vi "Get_Target_Type.vi"(8 "error in (no error)":errorcluster, 9 "install path":string, 10 "default install path":string, 11 "IB_Destination in":refnum<class "IB_Destination.lvclass">) -> (0 "error out":errorcluster, 1 "path for target type":T1=68 items=["Relative to default installation directory"=68, "Root directory on first partition"=70, "Relative to directory table key"=82, "Absolute path to file"=65], 2 "path for target":string, 3 "IB_Destination out":refnum<class "IB_Destination.lvclass">)   [LabVIEW 2020, in "IB_Destination.lvclass"]
uses:
  <vilib>/AppBuilder/IB_Classes/Destination/IB_Destination.lvclass
  <vilib>/AppBuilder/IB_Classes/Destination/IB_Destination.lvclass/IB_Destination.ctl
  AppLibs/distkit/MDF/NIMdf.llb/MDFBDPAddFilePathType.ctl
  AppLibs/distkit/MDF/NI_MDF.lvlib
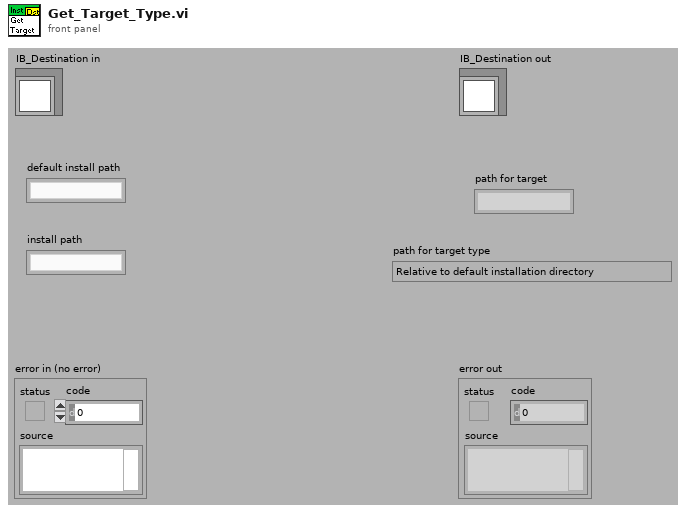
[diagram p1: front panel]
types:
  T1 = typedef "NI_MDF.lvlib/MDFBDPAddFilePathType.ctl" = i32
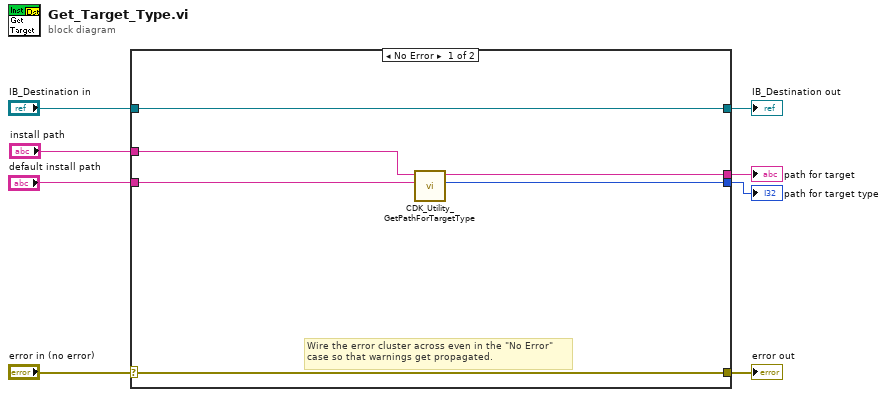
[diagram p0: block diagram]
diagram:
  n1 = case shown="No Error" "error in (no error)" {
    selector: "error in (no error)" -> [w14 w16]
    tunnel: [w14 w16] -> w7
    tunnel: [w13 w15] -> w5
    tunnel: "IB_Destination in" -> [w13 w15]
    tunnel: "default install path" -> [w12 _]
    tunnel: [w11 _] -> w3
    tunnel: [w10 _] -> w2
    tunnel: "install path" -> [w9 _]
    frame No Error {
      # "Wire the error cluster across even in the \"No Error\"\ncase so that warnings get propagated."
      n2 = call <resource>:"CDK_Utility_GetPathForTargetType.vi"("default install path"=w12, "eng_installPath"=w9) -> ("path for target type"=w10:T1, "path for target"=w11:string)  [unwired: 7 in, 1 out]
    }
    frame Error {
    }
  }
  "error out" <- w7
  "IB_Destination out" <- w5
  "path for target type" <- w2
  "path for target" <- w3
